vi "Next Cycle Globals.vi"() -> ()   [LabVIEW 2015, in "ECS-RT.lvlib"]
uses:
  ECS-RT.lvlib
  Typedefs/MISC/50% MFB - Results.ctl
  ECS-Shared.lvlib
panel:
  out "CA50 Control Output Valid":bool[](array[boolean])
  in  "Enable":bool
  out "CA50 Control Output [CAD]":sgl[](array[numeric]) format="%.2f"
  in  "Output Low [CAD]":sgl=-5.0 format="%.2f"
  in  "Output High [CAD]":sgl=5.0 format="%.2f"
  in  "D [min]":sgl format="%.3f"
  in  "I [min]":sgl=0.01 format="%.3f"
  in  "P":sgl=1.0 format="%.3f"
  in  "Setpoint [CAD]":sgl format="%.2f"
  in  "Timeout [ms]":u32=100
  out "CA50 Results":T1[](array[typedef])
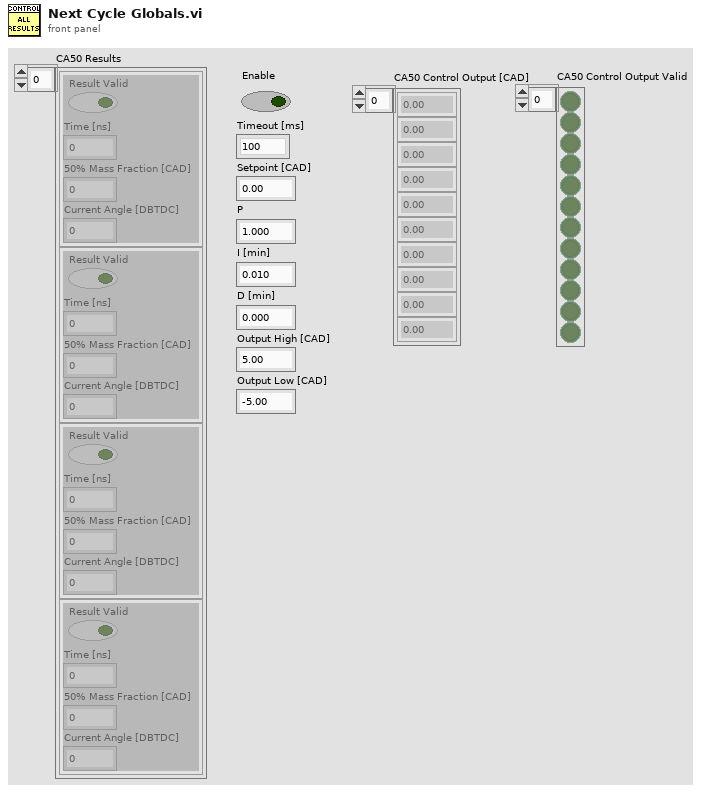
[diagram p1: front panel]
types:
  T1 = typedef "ECS-Shared.lvlib/50% MFB - Results.ctl" = cluster{"Result Valid":bool, "Time [ns]":u64, "50% Mass Fraction [CAD]":sgl, "Current Angle [DBTDC]":sgl}
diagram:
